vi "PauseMusicCommand_Create.vi"(0 "reference in":refnum<class "PauseMusicCommand.lvclass">, 5 "MediaPlayer":refnum<class "MediaPlayer.lvclass">, 11 "Error In":errorcluster) -> (4 "reference out":refnum<class "PauseMusicCommand.lvclass">, 15 "Error Out":errorcluster)   [LabVIEW 2024, in "PauseMusicCommand.lvclass"]
uses:
  PauseMusicCommand.lvclass
  Receiver/MediaPlayer_class/MediaPlayer.lvclass
panel:
  # "Connector Pane"
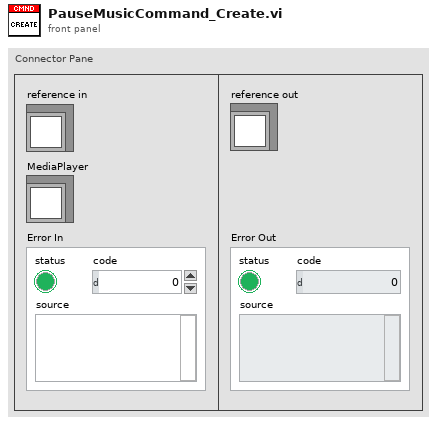
[diagram p1: front panel]
types:
  T1 = typedef "PauseMusicCommand.lvclass/ObjectAttributes.ctl" = cluster{"MediaPlayerRef":refnum<class "MediaPlayer.lvclass">}
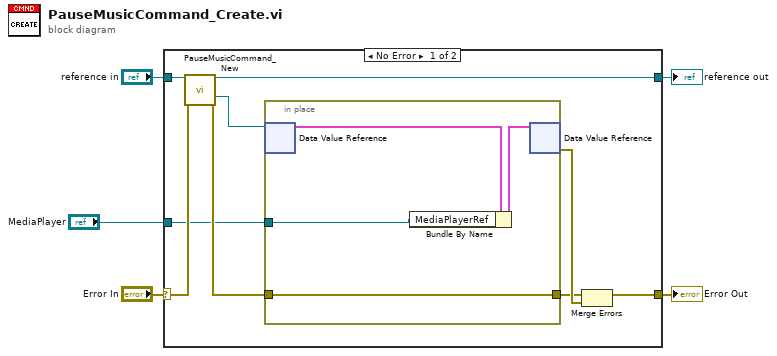
[diagram p0: block diagram]
diagram:
  n1 = case shown="No Error" "Error In" {
    selector: "Error In" -> [w13 w20]
    tunnel: [w7 w20] -> w4
    tunnel: "reference in" -> [w14 w19]
    tunnel: [w12 w19] -> w2
    tunnel: "MediaPlayer" -> [w6 _]
    frame No Error {
      n2 = call "PauseMusicCommand_New.vi"("reference in"=w14, "Error In"=w13) -> ("reference out"=w12:refnum<class "PauseMusicCommand.lvclass">, "DVRRefOut"=w10:refnum<data-value>, "Error Out"=w9:errorcluster)  [unwired: 10 in, 1 out]
      n3 = in-place {
        in-place-border: w9 -> [w16]
        in-place-border: [w16] -> w8
        in-place-border: w6 -> [w15]
        n4 = in-place-dvr #1(w10) -> (w17:T1)  [unwired: 1 out]
        n5 = Bundle By Name(cluster=w17, "MediaPlayerRef"=w15) -> (w18:T1)
        n6 = in-place-dvr #1(w18) -> (w11:errorcluster)  [unwired: 1 out]
      }
      n7 = Merge Errors(w8, w11) -> (w7:errorcluster)
    }
    frame Error {
      # "VI-TechBaseTemplate_Simple_4x4x4"
    }
  }
  "Error Out" <- w4
  "reference out" <- w2
